vi "数值二进制转十进制-8.6.vi"(4 "子数组":i32[](array[numeric])) -> (1 "十进制数值":i32)   [LabVIEW 2013]
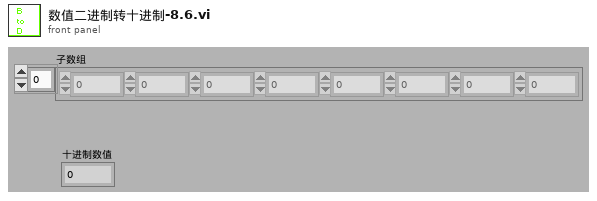
[diagram p1: front panel]
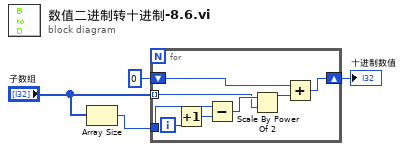
[diagram p0: block diagram]
diagram:
  n1 = Array Size(array="子数组") -> (size(s)=w3:i32)
  n2 = for {
    shift-right: [w10] -> w2
    shift-left: 0 -> [w12]
    tunnel: "子数组" -> [w5] mode=indexing
    tunnel: w3 -> [w8]
    i -> [w9]
    n3 = Increment(x=w9) -> (x+1=w7:i32)
    n4 = Subtract(x=w8, y=w7) -> (x-y=w6:i32)
    n5 = Scale By Power Of 2(n=w6, x=w5) -> (x*2^n=w11:i32)
    n6 = Add(x=w12, y=w11) -> (x+y=w10:i32)
  }
  "十进制数值" <- w2
